vi "Gain Tool Revised.vi"() -> ()   [LabVIEW 2018]
uses:
  <vilib>/DAQmx/write.llb/DAQmx Write (Digital Bool 1Line 1Point).vi
  <vilib>/DAQmx/read.llb/DAQmx Read (Analog DBL 1Chan 1Samp).vi
  <vilib>/DAQmx/create/channels.llb/DAQmx Create Channel (AI-Temperature-Thermocouple).vi
  <vilib>/DAQmx/miscellaneous.llb/DAQmx Fill In Error Info.vi
  <vilib>/DAQmx/create/channels.llb/DAQmx Create Channel (DO-Digital Output).vi
  <vilib>/addons/control/pid/pid.llb/PID Gain Schedule (DBL).vi
  <vilib>/addons/control/pid/autopid.llb/PID Online Autotuning (Step Closed Loop).vi
  <vilib>/addons/control/pid/pid.llb/PID Advanced (DBL).vi
  <vilib>/addons/control/pid/NI_PID_pid.lvlib
  <vilib>/ptbypt/NI_PtbyPt.lvlib
  <vilib>/addons/control/pid/NI_PID_autopid.lvlib
panel:
  in  "Sampling Time dt (s)":dbl=0.05 min=0.001 step=0.01 format="%#.3p"
  out "PV:":dbl(slide)=45.098041757771064 scale=0.0..100.0
  in  "Stop":bool
  out "SP and PV":cluster{"initial PV":dbl, "SP1:":dbl}(graph)={"initial PV"=50.98160323470328, "SP1:"=50.98039215686275}
  out "PID Gains":T1={"proportional gain (Kc)"=6.925505792902687, "integral time (Ti, min)"=0.004930412653813362, "derivative time (Td, min)"=0.0} {"derivative time (Td, min)" format="%#.6g"; "integral time (Ti, min)" format="%#.6g"; "proportional gain (Kc)" format="%#.6g"}
  in  "SP:":dbl(slide)=10.0 min=0.0 max=0.0 scale=0.0..100.0
  in  "MV:":dbl(slide)=-7.438794336301588e-06 scale=0.0..100.0
  in  "Autotune":bool
  in  "Replace gains":bool
  out "MV":dbl(graph)
  out "tuned PID gains":T1={"proportional gain (Kc)"=1.9838195929127882, "integral time (Ti, min)"=0.01995856284686879, "derivative time (Td, min)"=0.0} {"derivative time (Td, min)" format="%#.6g"; "integral time (Ti, min)" format="%#.6g"; "proportional gain (Kc)" format="%#.6g"}
  in  "autotuning parameters":T2={"Type of Controller"=1, "relay cycles"=3, "amplitude"=1.0, "control specifications"=2, "PV noise level"=0.1} {"PV noise level" format="%.2f"; "control specifications" items=["fast", "normal", "slow"]; "amplitude" format="%.2f"; "Type of Controller" items=["P", "PI", "PID"]}
  in  "Reinitialize":bool
  in  "Automatic":bool=TRUE
  in  "alpha":dbl=nan format="%.2f"
  in  "PID gain schedule":T3(array[cluster])=[{"PID gains"={"Kc"=7.0, "Ti"=0.001, "Td"=0.0}, "max value"=0.0}] {"max value" format="%.2f"; "PID gains"."Td" format="%#.3g"; "PID gains"."Ti" format="%#.3g"; "PID gains"."Kc" format="%#.3g"}
  in  "Insert gains":bool
  out "Gain Scheduling":i32
  # "Gain Scheduling"
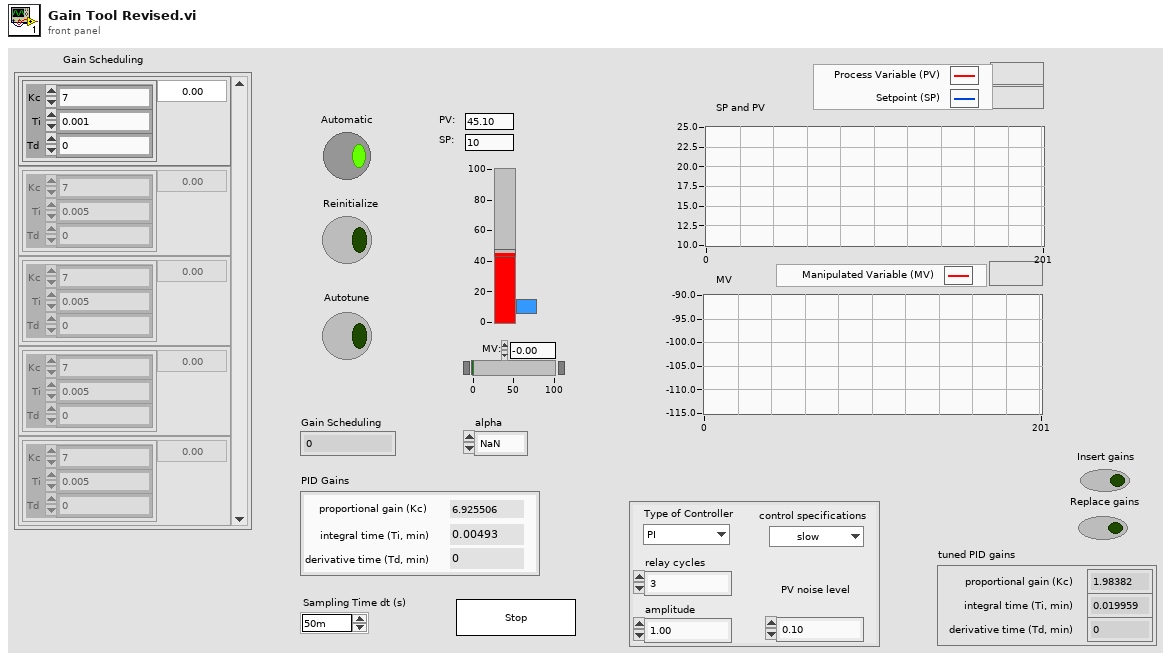
[diagram p1: front panel]
types:
  T1 = cluster{"proportional gain (Kc)":dbl, "integral time (Ti, min)":dbl, "derivative time (Td, min)":dbl}
  T2 = cluster{"Type of Controller":u16, "relay cycles":i32, "amplitude":dbl, "control specifications":u16, "PV noise level":dbl}
  T3 = cluster{"PID gains":cluster{"Kc":dbl, "Ti":dbl, "Td":dbl}, "max value":dbl}[]
  T4 = cluster{"tuned PID gains":cluster{"proportional gain (Kc)":dbl, "integral time (Ti, min)":dbl, "derivative time (Td, min)":dbl}, "SP:":dbl}
  T5 = cluster{"PID gains":cluster{"Kc":dbl, "Ti":dbl, "Td":dbl}, "max value":dbl}
  T6 = cluster{"tuned PID gains":cluster{"proportional gain (Kc)":dbl, "integral time (Ti, min)":dbl, "derivative time (Td, min)":dbl}, "max value":dbl}
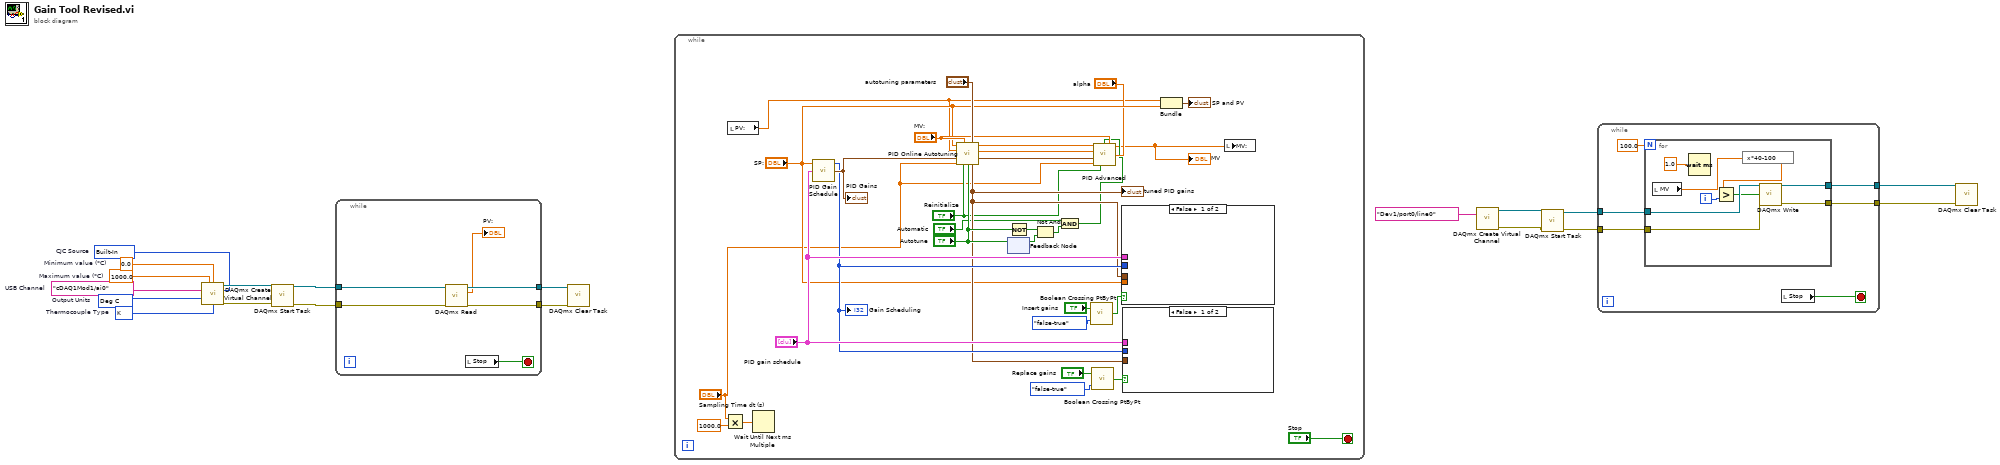
[diagram p0: block diagram]
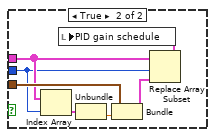
[diagram p2: hidden frame]
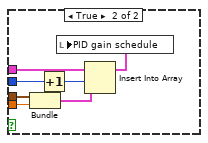
[diagram p3: hidden frame]
diagram:
  w11 = 10143 items=["Deg C"=10143, "Deg F"=10144, "Kelvins"=10325, "Deg R"=10145, "From Custom Scale"=10065]  # Output Units
  w15 = 10073 items=["J"=10072, "K"=10073, "N"=10077, "R"=10082, "S"=10085, "T"=10086, "B"=10047, "E"=10055]  # Thermocouple Type
  w12 = tag "cDAQ1Mod1/ai0"  # USB Channel
  w13 = 1000.0  # Maximum value (*C)
  w14 = 0.0  # Minimum value (*C)
  w10 = 10200 items=["Built-In"=10200, "Constant Value"=10116, "Channel"=10113]  # CJC Source
  n1 = call-poly <vilib>:"DAQmx Create Virtual Channel.vi"("maximum value"=w13, "minimum value"=w14, "physical channels"=w12, "cjc source"=w10, "units"=w11, "thermocouple type"=w15) -> ("task out"=w19:refnum<k21>, "error out"=w17:errorcluster)  [unwired: 8 in]
  n2 = call <vilib>:"DAQmx Start Task.vi"("task/channels in"=w19, "error in"=w17) -> ("task out"=w18:refnum<k21>, "error out"=w16:errorcluster)  [unwired: 12 in]
  n3 = while {
    tunnel: w18 -> [w25]
    tunnel: w16 -> [w24]
    tunnel: [w23] -> w9
    tunnel: [w22] -> w8
    stop <- w20 stop-if-true
    n4 = call-poly <vilib>:"DAQmx Read.vi"("task/channels in"=w25, "error in"=w24) -> ("task out"=w23:refnum<k21>, "data"=→"PV:":dbl, "error out"=w22:errorcluster)  [unwired: 11 in]
    n5 = local read "Stop"() -> (w20:bool)
  }
  n6 = call <vilib>:"DAQmx Clear Task.vi"("task in"=w9, "error in"=w8) -> ()  [unwired: 13 in, 1 out]
  n7 = while {
    stop <- "Stop" stop-if-true
    n8 = Multiply(x="Sampling Time dt (s)", y=1000.0) -> (x*y=w29:dbl)
    n9 = local read "PV:"() -> (w31:dbl)
    n10 = Wait Until Next ms Multiple(millisecond multiple=w29) -> ()  [unwired: 1 out]
    n11 = call-poly <vilib>:"PID Gain Schedule.vi"("PID gain schedule"="PID gain schedule", "gain scheduling value"="SP:") -> ("PID gains out"=w44:T1, "index out"=w39:i32)  [unwired: 2 in]
    "PID Gains" <- w44
    "Gain Scheduling" <- w39
    n12 = call-poly <vilib>:"PID Online Autotuning.vi"("setpoint"="SP:", "manipulated variable"="MV:", "autotuning parameters"="autotuning parameters", "process variable"=w31, "PID gains in"=w44, "dt (s)"="Sampling Time dt (s)", "reinitialize? (F)"="Reinitialize", "autotune? (F)"="Autotune") -> ("setpoint out"=w55:dbl, "process variable out"=w54:dbl, "PID gains out"=w52:T1, "tuned PID gains"=w38:T1)  [unwired: 3 in, 1 out]
    "tuned PID gains" <- w38
    n13 = feedback #1() -> (w50:bool)  [unwired: 1 in]
    n14 = feedback-in #1("Autotune") -> ()
    n15 = Not(x="Autotune") -> (.not. x?=w47:bool)
    n16 = Not And(1:w50, 2:w47) -> (0:w48:bool)
    n17 = And(x="Automatic", y=w48) -> (x .and. y?=w34:bool)
    n18 = call <vilib>:"Boolean Crossing PtByPt.vi"("direction"=enum16{"either", "false-true", "true-false"}."false-true", "input"="Insert gains") -> ("crossing"=w45:bool)  [unwired: 1 in]
    n19 = call <vilib>:"Boolean Crossing PtByPt.vi"("direction"=enum16{"either", "false-true", "true-false"}."false-true", "input"="Replace gains") -> ("crossing"=w41:bool)  [unwired: 1 in]
    n20 = call-poly <vilib>:"PID Advanced.vi"("setpoint"=w55, "auto? (T)"=w34, "manual control"="MV:", "process variable"=w54, "alpha"="alpha", "PID gains"=w52, "dt (s)"="Sampling Time dt (s)", "reinitialize? (F)"="Reinitialize") -> ("output"=w26:dbl)  [unwired: 6 in, 1 out]
    "MV" <- w26
    n21 = case shown="False" w45 {
      tunnel: w38 -> [_ w70]
      tunnel: "SP:" -> [_ w69]
      tunnel: "PID gain schedule" -> [_ w67]
      tunnel: w39 -> [_ w65]
      frame False {
      }
      frame True {
        n22 = Bundle("tuned PID gains"=w70, "SP:"=w69) -> (w68:T4)  [unwired: 1 in]
        n23 = Increment(x=w65) -> (x+1=w64:i32)
        n24 = Insert Into Array(array=w67, index=w64, new element=w68) -> (w66:T3)
        n25 = local write "PID gain schedule"(w66) -> ()
      }
    }
    n26 = case shown="False" w41 {
      tunnel: w38 -> [_ w63]
      tunnel: "PID gain schedule" -> [_ w60]
      tunnel: w39 -> [_ w59]
      frame False {
      }
      frame True {
        n27 = Index Array(array=w60, index=w59) -> (element=w58:T5)
        n28 = Unbundle(w58) -> ("max value"=w57:dbl)  [unwired: 1 out]
        n29 = Bundle("tuned PID gains"=w63, "max value"=w57) -> (w61:T6)  [unwired: 1 in]
        n30 = Replace Array Subset(array=w60, new element=w61, index=w59) -> (w62:T3)
        n31 = local write "PID gain schedule"(w62) -> ()
      }
    }
    n32 = Bundle("PV:"=w31, "SP:"="SP:") -> (→"SP and PV":cluster{"PV: ":dbl, "SP:":dbl})  [unwired: 1 in]
    n33 = local write "MV:"(w26) -> ()
  }
  n34 = call-poly <vilib>:"DAQmx Create Virtual Channel.vi"("lines"=tag "Dev1/port0/line0") -> ("task out"=w5:refnum<k21>, "error out"=w4:errorcluster)  [unwired: 13 in]
  n35 = call <vilib>:"DAQmx Start Task.vi"("task/channels in"=w5, "error in"=w4) -> ("task out"=w3:refnum<k21>, "error out"=w2:errorcluster)  [unwired: 12 in]
  n36 = while {
    tunnel: [w75] -> w7
    tunnel: [w74] -> w6
    tunnel: w3 -> [w73]
    tunnel: w2 -> [w72]
    stop <- w71 stop-if-true
    n37 = for {
      N: 100.0 -> [_]
      tunnel: [w83] -> w75
      tunnel: [w82] -> w74
      tunnel: w73 -> [w81]
      tunnel: w72 -> [w80]
      i -> [w85]
      n38 = local read "MV"() -> (w79:dbl)
      n39 = Wait (ms)(milliseconds to wait=1.0) -> ()  [unwired: 1 out]
      n40 = expression code="x*40-100"(w79) -> (w78:dbl)
      n41 = Greater?(x=w78, y=w85) -> (0:w77:bool)
      n42 = call-poly <vilib>:"DAQmx Write.vi"("task/channels in"=w81, "data"=w77, "error in"=w80) -> ("task out"=w83:refnum<k21>, "error out"=w82:errorcluster)  [unwired: 10 in, 1 out]
    }
    n43 = local read "Stop"() -> (w71:bool)
  }
  n44 = call <vilib>:"DAQmx Clear Task.vi"("task in"=w7, "error in"=w6) -> ()  [unwired: 13 in, 1 out]
